vi "shift odd lines by.vi"(5 "calculate squared difference":bool, 7 "shift odd lines by":i32, 8 "max pix shift":i32=150, 11 "frame in":dbl[][](array[numeric])) -> (2 "squared difference":dbl, 3 "shifted frame out":dbl[][](array[numeric]))   [LabVIEW 2012]
doc: "SciScan 1.2 160622"
panel:
  out "corrected 3":T1(plugin-control)
  out "corrected 2":T1(plugin-control)
  out "size(s) 7":i32[](array[numeric])
  out "size(s) 6":i32[](array[numeric])
  out "size(s) 5":i32[](array[numeric])
  out "size(s) 4":i32
  out "size(s) 3":i32[](array[numeric])
  out "size(s) 2":i32[](array[numeric])
  out "size(s)":i32[](array[numeric])
  in  "display on/off":bool
  out "corrected":T1(plugin-control)
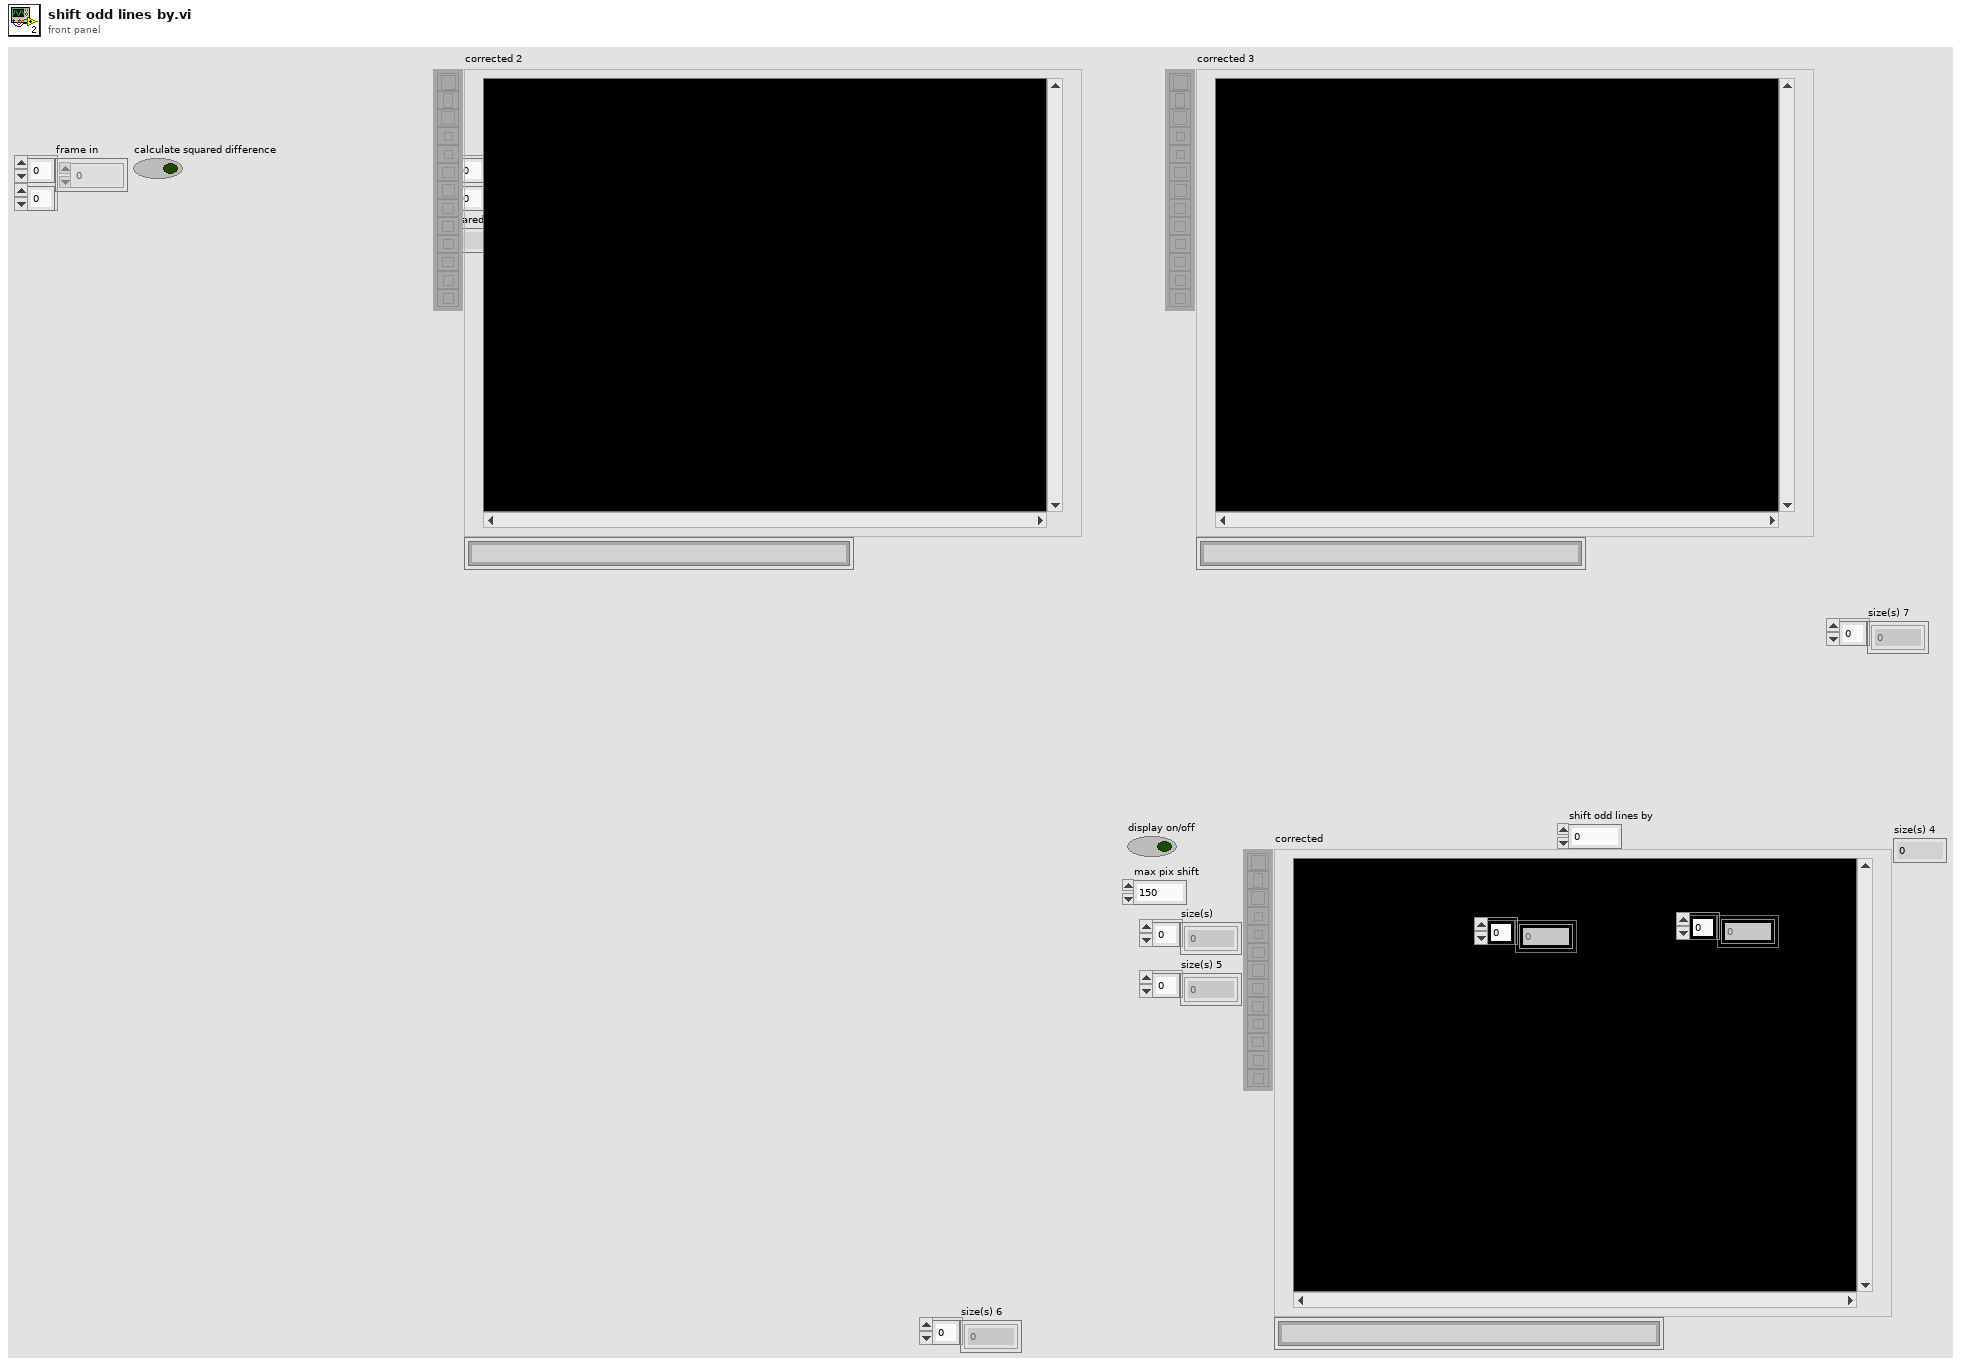
[diagram p1: front panel]
types:
  T1 = typedef "IMAQ Image.ctl" = refnum<image>
  T2 = typedef "Image Type" = u32
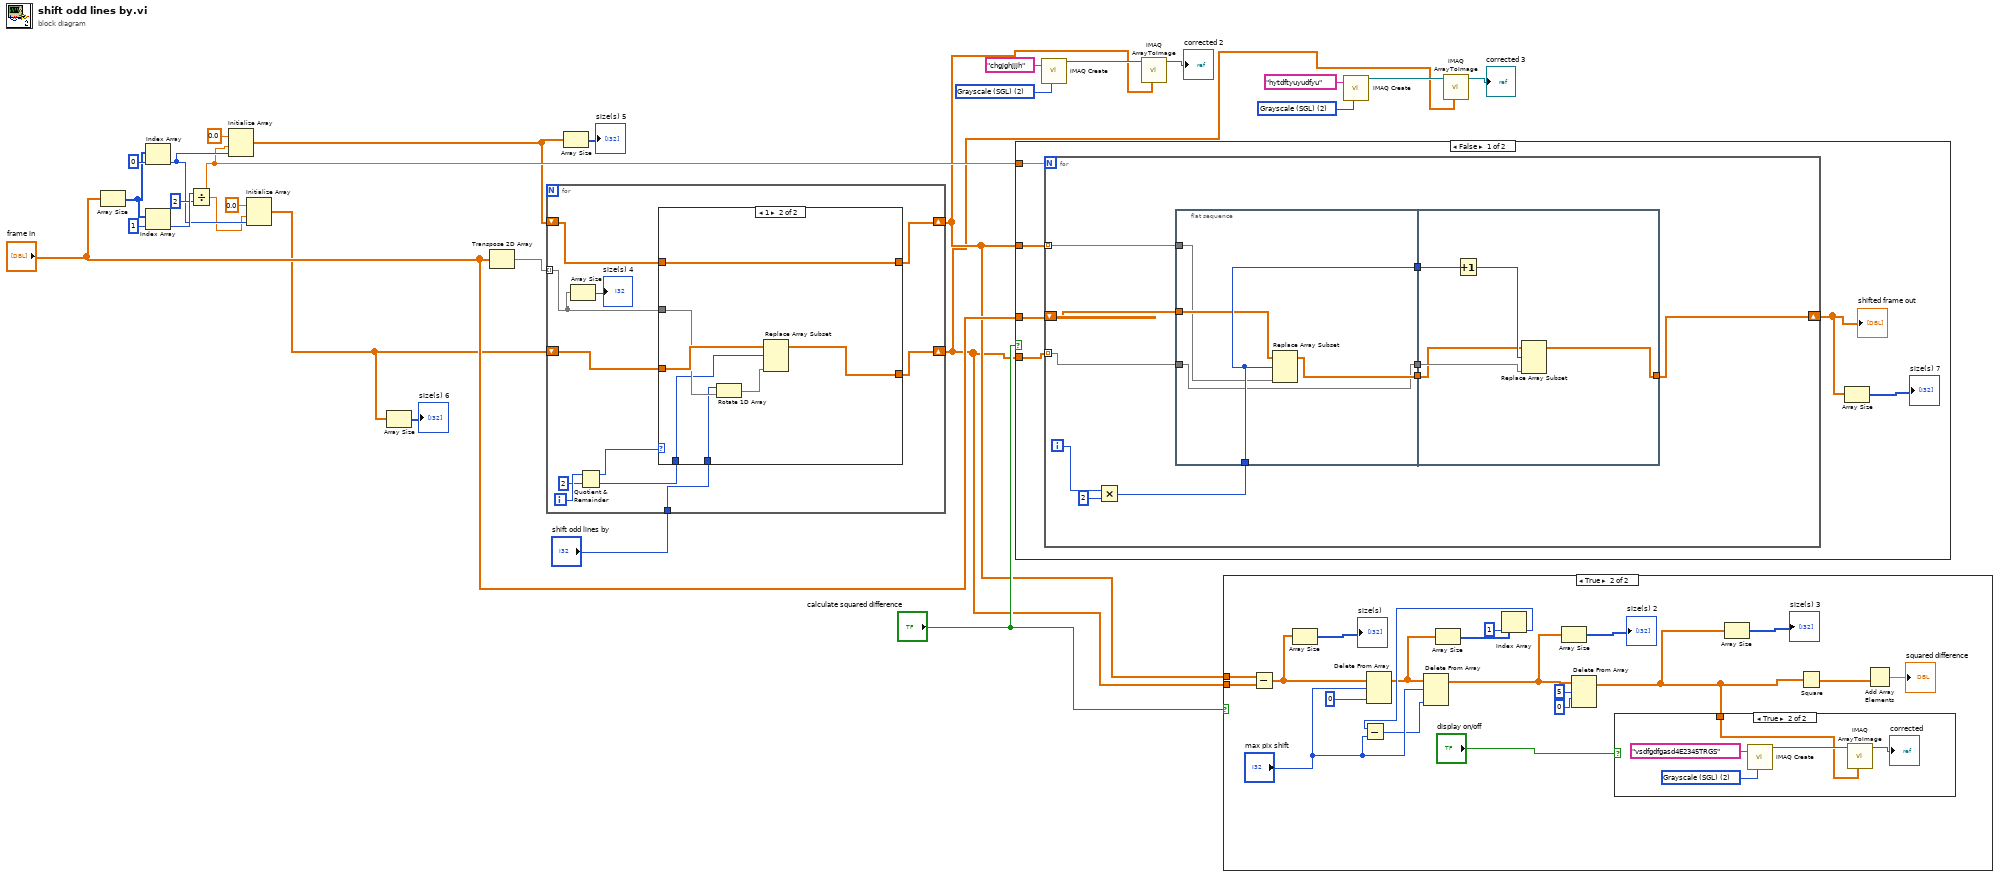
[diagram p0: block diagram]
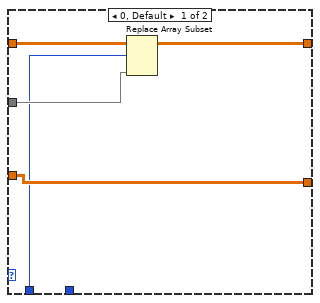
[diagram p5: hidden frame]
diagram:
  w6 = T2 2 items=["Grayscale (U8)", "Grayscale (I16)", "Grayscale (SGL)", "Complex (CSG)", "RGB (U32)", "HSL (U32)", "RGB (U64)", "Grayscale (U16)"] ("Image Type")
  w7 = T2 2 items=["Grayscale (U8)", "Grayscale (I16)", "Grayscale (SGL)", "Complex (CSG)", "RGB (U32)", "HSL (U32)", "RGB (U64)", "Grayscale (U16)"] ("Image Type")
  n1 = Array Size(array="frame in") -> (size(s)=w25:i32[])
  n2 = Index Array(array=w25, index=0) -> (element=w19:i32)
  n3 = Index Array(array=w25, index=1) -> (element=w24:i32)
  n4 = Divide(x=w24, y=2) -> (x/y=w18:dbl)
  n5 = Initialize Array(0.0 ("element"), w18, w19) -> (w15:dbl[][])
  n6 = Initialize Array(0.0 ("element"), w18, w19) -> (w12:dbl[][])
  n7 = Array Size(array=w12) -> (size(s)=→"size(s) 6":i32[])
  n8 = Transpose 2D Array(2D array="frame in") -> (transposed array=w11:dbl[][])
  n9 = for {
    tunnel: w11 -> [w29] mode=indexing
    shift-right: [w34] -> w2
    shift-left: w15 -> [w35]
    shift-right: [w31] -> w1
    shift-left: w12 -> [w32]
    tunnel: "shift odd lines by" -> [w30]
    i -> [w38]
    n10 = Array Size(array=w29) -> (size(s)=→"size(s) 4":i32)
    n11 = Quotient & Remainder(x=w38, y=2) -> (x-y*floor(x/y)=w36:i32, floor(x/y)=w33:i32)
    n12 = case shown="1" w36 {
      tunnel: w29 -> [w41 w49]
      tunnel: w35 -> [w43 w46]
      tunnel: [w42 w46] -> w34
      tunnel: w33 -> [w39 w44]
      tunnel: w32 -> [w40 w50]
      tunnel: [w40 w47] -> w31
      tunnel: w30 -> [_ w45]
      frame 0, Default {
        n13 = Replace Array Subset(array=w43, new element=w41, index (row)=w39) -> (w42:dbl[][])  [unwired: 1 in]
      }
      frame 1 {
        n14 = Rotate 1D Array(1:w49, 2:w45) -> (0:w48:dbl[])
        n15 = Replace Array Subset(array=w50, new element=w48, index (row)=w44) -> (w47:dbl[][])  [unwired: 1 in]
      }
    }
  }
  n16 = Array Size(array=w15) -> (size(s)=→"size(s) 5":i32[])
  n17 = case shown="False" "calculate squared difference" {
    tunnel: "frame in" -> [w56 _]
    tunnel: w2 -> [w55 _]
    tunnel: w1 -> [w54 _]
    tunnel: w18 -> [w53 _]
    frame False {
      n18 = for {
        N: w53 -> [_]
        shift-right: [w62] -> w51
        shift-left: w56 -> [w66]
        tunnel: w55 -> [w63] mode=indexing
        tunnel: w54 -> [w65] mode=indexing
        i -> [w64]
        n19 = Multiply(x=w64, y=2) -> (x*y=w61:i32)
        n20 = flat-sequence {
          tunnel: w66 -> [w70]
          tunnel: [w68] -> w59
          tunnel: w65 -> [w67]
          tunnel: [w67] -> w58
          tunnel: w61 -> [w71]
          tunnel: [w71] -> w57
          tunnel: w63 -> [w69]
          tunnel: [w73] -> w62
          tunnel: w59 -> [w72]
          tunnel: w58 -> [w76]
          tunnel: w57 -> [w75]
          frame #0 {
            n21 = Replace Array Subset(array=w70, new element=w69, index (row)=w71) -> (w68:dbl[][])  [unwired: 1 in]
          }
          frame #1 {
            n22 = Increment(x=w75) -> (x+1=w74:i32)
            n23 = Replace Array Subset(array=w72, new element=w76, index (row)=w74) -> (w73:dbl[][])  [unwired: 1 in]
          }
        }
      }
      "shifted frame out" <- w51
      n24 = Array Size(array=w51) -> (size(s)=→"size(s) 7":i32[])
    }
    frame True {
    }
  }
  n25 = call "IMAQ Create"("Image Name"="chgjghjjjh", "Image Type"=w7) -> ("New Image"=w9:T1)  [unwired: 3 in, 1 out]
  n26 = call "IMAQ ArrayToImage"("Image Pixels (Float)"=w2, "Image"=w9) -> ("Image Out"=→"corrected 2":T1)  [unwired: 8 in, 1 out]
  n27 = case shown="True" "calculate squared difference" {
    tunnel: w2 -> [_ w95]
    tunnel: w1 -> [_ w94]
    frame False {
    }
    frame True {
      n28 = Subtract(x=w95, y=w94) -> (x-y=w85:dbl[][])
      n29 = Array Size(array=w85) -> (size(s)=→"size(s)":i32[])
      n30 = Delete From Array(array=w85, length="max pix shift", index (col)=0 ("index (row)")) -> (array with subset deleted=w89:dbl[][])  [unwired: 1 in, 1 out]
      n31 = Array Size(array=w89) -> (size(s)=w92:i32[])
      n32 = Index Array(array=w92, index=1) -> (element=w90:i32)
      n33 = Subtract(x=w90, y="max pix shift") -> (x-y=w78:i32)
      n34 = Delete From Array(array=w89, length="max pix shift", index (col)=w78) -> (array with subset deleted=w82:dbl[][])  [unwired: 1 in, 1 out]
      n35 = Array Size(array=w82) -> (size(s)=→"size(s) 2":i32[])
      n36 = Delete From Array(array=w82, length=5, index (row)=0) -> (array with subset deleted=w80:dbl[][])  [unwired: 1 in, 1 out]
      n37 = case shown="True" "display on/off" {
        tunnel: w80 -> [_ w97]
        frame False {
        }
        frame True {
          w101 = T2 2 items=["Grayscale (U8)", "Grayscale (I16)", "Grayscale (SGL)", "Complex (CSG)", "RGB (U32)", "HSL (U32)", "RGB (U64)", "Grayscale (U16)"] ("Image Type")
          n38 = call "IMAQ Create"("Image Name"="vsdfgdfgasd4E2345TRGS", "Image Type"=w101) -> ("New Image"=w99:T1)  [unwired: 3 in, 1 out]
          n39 = call "IMAQ ArrayToImage"("Image Pixels (Float)"=w97, "Image"=w99) -> ("Image Out"=→"corrected":T1)  [unwired: 8 in, 1 out]
        }
      }
      n40 = Array Size(array=w80) -> (size(s)=→"size(s) 3":i32[])
      n41 = Square(x=w80) -> (x^2=w96:dbl[][])
      n42 = Add Array Elements(numeric array=w96) -> (sum=→"squared difference":dbl)
    }
  }
  n43 = call "IMAQ Create"("Image Name"="hytdftyuyudfyu", "Image Type"=w6) -> ("New Image"=w4:T1)  [unwired: 3 in, 1 out]
  n44 = call "IMAQ ArrayToImage"("Image Pixels (Float)"=w1, "Image"=w4) -> ("Image Out"=→"corrected 3":T1)  [unwired: 8 in, 1 out]
